vi "p1.vi"() -> ()   [LabVIEW 2025, in "d10.lvlib"]
uses:
  d10.lvlib
  <vilib>/Utility/miscctls.llb/LVMapReplaceAction.ctl
  AOC/AOC.lvlib
  <userlib>/_OpenG.lib/string/string.llb/openg_string.lvlib
panel:
  out "Answer":u64
  in  "Example":string="[.##.] (3) (1,3) (2) (2,3) (0,2) (0,1) {3,5,4,7}\n[...#.] (0,2,3,4) (2,3) (0,4) (0,1,2) (1,2,3,4) {7,5,12,7,2}\n[.###.#] (0,1,2,3,4) (0,3,4) (0,1,2,4,5) (1,2) {10,11,11,5,10,5}"
  in  "Example":bool=TRUE
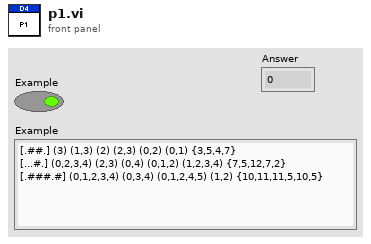
[diagram p1: front panel]
types:
  T1 = typedef "LVMapReplaceAction.ctl" = enum32{"Modify Entry only if found", "Add or Modify Entry", "Delete Entry"}
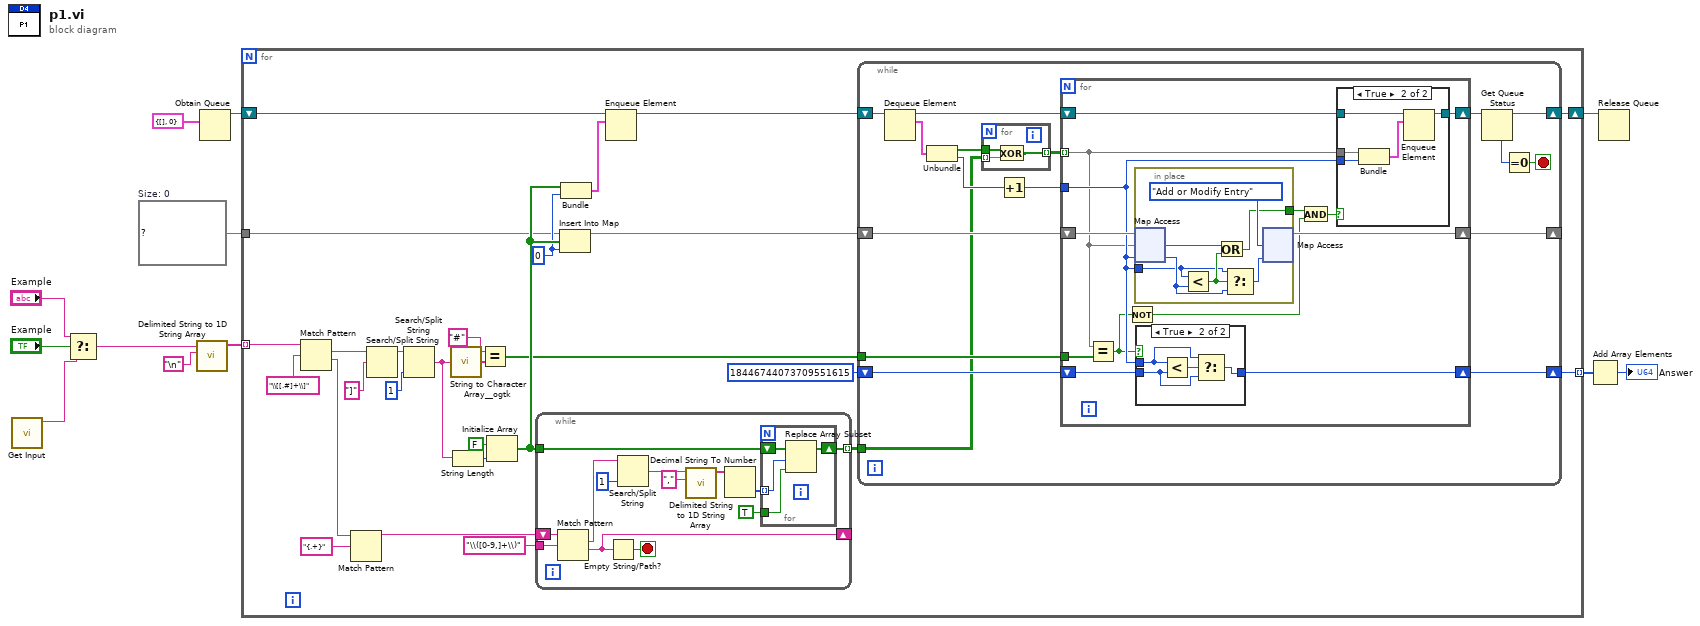
[diagram p0: block diagram]
diagram:
  w5 = map{bool[], u64} {}  # Size: 0
  n1 = call "Get Input.vi"() -> ("Input"=w12:string)  [unwired: 11 in]
  n2 = Select(t="Example", s="Example", f=w12) -> (s? t:f=w1:string)
  n3 = call <vilib>:"Delimited String to 1D String Array.vi"("delimiter"="\n", "delimited string"=w1) -> ("string array"=w8:string[])  [unwired: 9 in]
  n4 = Obtain Queue(element data type=cluster{bool[], u64} {[], 0} ("output cluster")) -> (queue out=w3:refnum<queue>)  [unwired: 4 in, 2 out]
  n5 = for {
    tunnel: w8 -> [w39] mode=indexing
    tunnel: [w23] -> w7 mode=indexing
    tunnel: w5 -> [w19]
    shift-right: [w13] -> w2
    shift-left: w3 -> [w15]
    w24 = u64 0
    n6 = Match Pattern(string=w39, regular expression="\\[[.#]+\\]") -> (match substring=w37:string, after substring=w38:string)  [unwired: 1 in, 2 out]
    n7 = Match Pattern(string=w38, regular expression="{.+}") -> (before substring=w33:string)  [unwired: 1 in, 3 out]
    n8 = Search/Split String(string=w37, search string/char (-)="]") -> (substring before match=w32:string)  [unwired: 1 in, 2 out]
    n9 = Search/Split String(string=w32, offset (0)=1) -> (match + rest of string=w22:string)  [unwired: 1 in, 2 out]
    n10 = call <userlib>:"String to Character Array__ogtk.vi"("Input String"=w22) -> ("Character Array"=w21:string[])
    n11 = String Length(string=w22) -> (length=w20:i32)
    n12 = Equal?(x="#", y=w21) -> (x = y?=w29:bool[])
    n13 = Initialize Array(FALSE, w20) -> (w30:bool[])
    n14 = while {
      shift-right: [w92] -> _
      shift-left: w33 -> [w95]
      tunnel: w30 -> [w102]
      tunnel: [w96] -> w26 mode=indexing
      tunnel: "\\([0-9,]+\\)" ("regular expression") -> [w94]
      stop <- w97 stop-if-true
      n15 = Match Pattern(string=w95, regular expression=w94) -> (match substring=w93:string, after substring=w92:string)  [unwired: 1 in, 2 out]
      n16 = Empty String/Path?(string/path=w92) -> (empty?=w97:bool)
      n17 = Search/Split String(string=w93, offset (0)=1) -> (match + rest of string=w98:string)  [unwired: 1 in, 2 out]
      n18 = call <vilib>:"Delimited String to 1D String Array.vi"("delimiter"=",", "delimited string"=w98) -> ("string array"=w101:string[])  [unwired: 9 in]
      n19 = Decimal String To Number(string=w101) -> (number=w100:i32[])  [unwired: 2 in, 1 out]
      n20 = for {
        shift-right: [w105] -> w96
        shift-left: w102 -> [w107]
        tunnel: w100 -> [w106] mode=indexing
        tunnel: TRUE ("new element/subarray") -> [w104]
        n21 = Replace Array Subset(array=w107, new element=w104, index=w106) -> (w105:bool[])
      }
    }
    n22 = Insert Into Map(map in=w19, key=w30, value=w24) -> (map out=w25:map{bool[], u64})  [unwired: 2 out]
    n23 = Bundle(w30, w24) -> (w28:cluster{bool[], u64})  [unwired: 1 in]
    n24 = Enqueue Element(queue=w15, element=w28) -> (queue out=w27:refnum<queue>)  [unwired: 2 in, 2 out]
    n25 = while {
      shift-right: [w49] -> _
      shift-left: w25 -> [w51]
      tunnel: w26 -> [w46]
      tunnel: w29 -> [w52]
      shift-right: [w50] -> w23
      shift-left: u64 18446744073709551615 -> [w53]
      shift-right: [w42] -> w13
      shift-left: w27 -> [w56]
      stop <- w40 stop-if-true
      n26 = Dequeue Element(queue=w56) -> (queue out=w47:refnum<queue>, element=w55:cluster{bool[], u64})  [unwired: 2 in, 2 out]
      n27 = Unbundle(w55) -> (w45:bool[], w54:u64)
      n28 = for {
        tunnel: w46 -> [w90] mode=indexing
        tunnel: w45 -> [w89]
        tunnel: [w88] -> w44 mode=indexing
        n29 = Exclusive Or(1:w90, 2:w89) -> (0:w88:bool[])
      }
      n30 = Increment(x=w54) -> (x+1=w48:u64)
      n31 = for {
        shift-right: [w65] -> w50
        shift-left: w53 -> [w66]
        tunnel: w52 -> [w67]
        shift-right: [w68] -> w49
        shift-left: w51 -> [w69]
        tunnel: w44 -> [w57] mode=indexing
        tunnel: w48 -> [w61]
        shift-right: [w64] -> w43
        shift-left: w47 -> [w63]
        n32 = Equal?(x=w57, y=w67) -> (x = y?=w59:bool)
        n33 = Not(x=w59) -> (.not. x?=w58:bool)
        n34 = in-place {
          in-place-border: w61 -> [w70]
          in-place-border: [w71] -> w62
          n35 = in-place-map #1(w69, w57, w61) -> (w75:u64, w72:bool)
          n36 = Less?(x=w70, y=w75) -> (x < y?=w73:bool)
          n37 = Or(x=w72, y=w73) -> (x .or. y?=w71:bool)
          n38 = Select(t=w70, s=w73, f=w75) -> (s? t:f=w76:u64)
          n39 = in-place-map #1(w76, LVMapReplaceAction."Add or Modify Entry" ("action")) -> (w68:map{bool[], u64})  [unwired: 2 out]
        }
        n40 = case shown="True" w59 {
          tunnel: w66 -> [w77 w80]
          tunnel: w61 -> [_ w81]
          tunnel: [w77 w79] -> w65
          frame False {
          }
          frame True {
            n41 = Less?(x=w81, y=w80) -> (x < y?=w78:bool)
            n42 = Select(t=w81, s=w78, f=w80) -> (s? t:f=w79:u64)
          }
        }
        n43 = And(x=w62, y=w58) -> (x .and. y?=w60:bool)
        n44 = case shown="True" w60 {
          tunnel: [w82 w87] -> w64
          tunnel: w63 -> [w82 w86]
          tunnel: w57 -> [_ w85]
          tunnel: w61 -> [_ w84]
          frame False {
          }
          frame True {
            n45 = Bundle(w85, w84) -> (w83:cluster{bool[], u64})  [unwired: 1 in]
            n46 = Enqueue Element(queue=w86, element=w83) -> (queue out=w87:refnum<queue>)  [unwired: 2 in, 2 out]
          }
        }
      }
      n47 = Get Queue Status(queue=w43) -> (queue out=w42:refnum<queue>, # elements in queue=w41:i32)  [unwired: 2 in, 6 out]
      n48 = Equal To 0?(x=w41) -> (x = 0?=w40:bool)
    }
  }
  n49 = Add Array Elements(numeric array=w7) -> (sum=→"Answer":u64)
  n50 = Release Queue(queue=w2) -> ()  [unwired: 2 in, 3 out]
